vi "WriteToBaseConfigVariant.vi"(6 "Measurement Refresh Time (ms)":u32, 8 "error in (no error)":errorcluster, 9 "Meas":variant, 10 "Config":variant, 11 "NHRDCModel in":refnum<class "NHRDCModel.lvclass">) -> (0 "error out":errorcluster, 3 "NHRDCModel out":refnum<class "NHRDCModel.lvclass">)   [LabVIEW 2018, in "AcPwrPlugins.lvlib" / "NHRDCModel.lvclass"]
uses:
  NHRDCModel.lvclass
  AcPwrBaseClass/AcPwrBase.lvclass
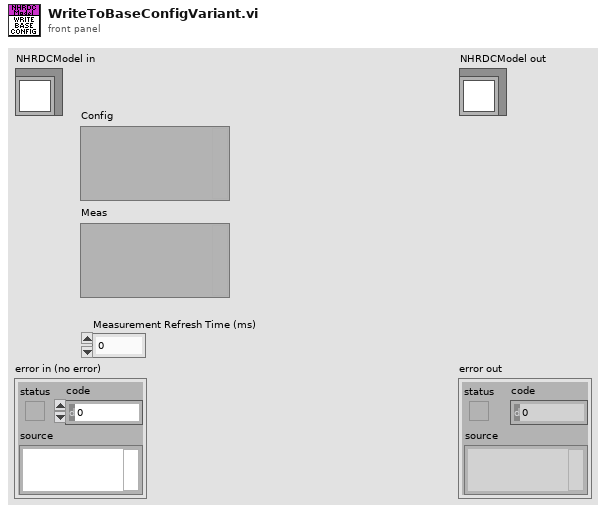
[diagram p1: front panel]
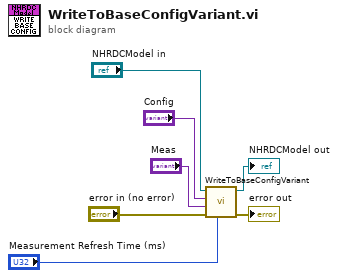
[diagram p0: block diagram]
diagram:
  n1 = call-parent "WriteToBaseConfigVariant.vi"("Measurement Refresh Time (ms)"="Measurement Refresh Time (ms)", "error in (no error)"="error in (no error)", "Meas"="Meas", "Config"="Config", "AcPwrBase in"="NHRDCModel in") -> ("error out"=→"error out":errorcluster, "AcPwrBase out"=→"NHRDCModel out":refnum<class "NHRDCModel.lvclass">)  [unwired: 5 in]
